vi "Alicat Simplified Driver Example.vi"() -> ()   [LabVIEW 2019]
doc: "Simplified example program for initializing the COM port, determining the data frame of an Alicat, and acquiring the data of the same Alicat.\n\nThis is intended to be a good starting point for either creating a new program or integrating Alicat devices with an existing program."
uses:
  Sub-VIs/Data Cluster.ctl
panel:
  out "Measurement Data":T1
  in  "Minimum time \nbetween readings [ms]":u32
  out "Measurements\nper second":dbl
  in  "End Program":bool
  out "Error Text":string
  out "Error Present":bool
  out "Range Exceeded":bool
  in  "COM Port Settings":T2={"Unit ID"="A", "Baud Rate"=enum."19200", "VISA Sesssion In"="COM1"}
  # "Totalizer Timer"
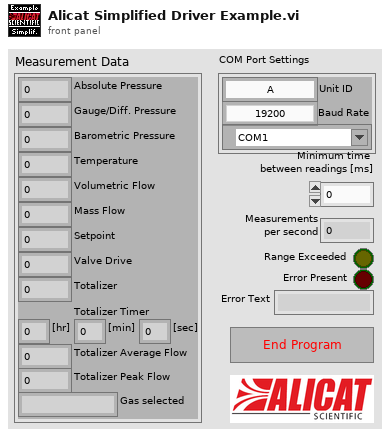
[diagram p1: front panel]
types:
  T1 = typedef "Data Cluster.ctl" = cluster{"Absolute Pressure":dbl, "Gauge/Diff. Pressure":dbl, "Barometric Pressure":dbl, "Temperature":dbl, "Volumetric Flow":dbl, "Mass Flow":dbl, "Setpoint":dbl, "Valve Drive":dbl, "Totalizer":dbl, "[hr]":dbl, "[min]":dbl, "[sec]":dbl, "Totalizer Average Flow":dbl, "Totalizer Peak Flow":dbl, "Gas selected":string}
  T2 = cluster{"Unit ID":string, "Baud Rate":enum8{"2400", "9600", "19200", "38400", "57600", "115200", "Unknown"}, "VISA Sesssion In":refnum<visa-resource-name>}
  T3 = typedef "Data Frame.ctl" = cluster{"Absolute Pressure":bool, "Gauge/Diff. Pressure":bool, "Barometric Pressure":bool, "Temperature":bool, "Volumetric":bool, "Mass":bool, "Setpoint":bool, "Valve Drive":bool, "Totalizer":bool, "Totalizer Timer":bool, "Totalizer Average Flow":bool, "Totalizer Peak Flow":bool, "Gas Selected":bool, "Tot. Timer Format":u16}
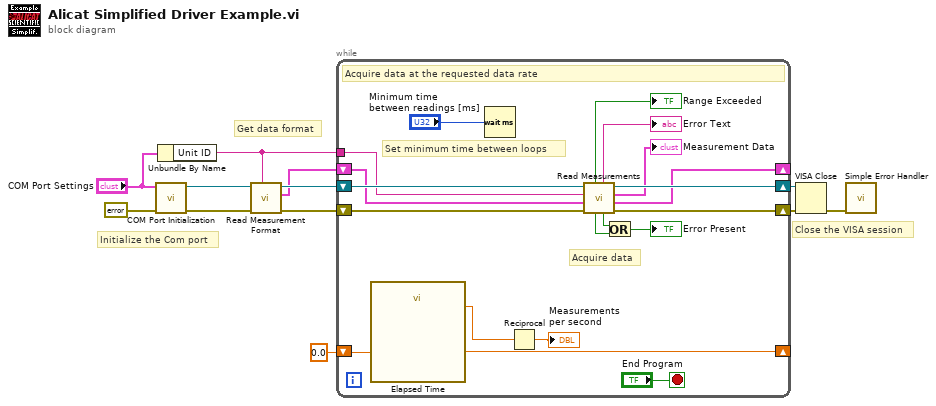
[diagram p0: block diagram]
diagram:
  # "Get data format"
  # "Close the VISA session"
  # "Initialize the Com port"
  n1 = call "COM Port Initialization.vi"("error in (no error)"=errorcluster {"status"=FALSE, "code"=0, "source"=""}, "Communication Settings"="COM Port Settings") -> ("error out"=w6:errorcluster, "VISA Session Out"=w5:refnum<visa-resource-name>)  [unwired: 8 in]
  n2 = Unbundle By Name("COM Port Settings") -> ("Unit ID"=w1:string)
  n3 = call "Read Measurement Format.vi"("Unit ID (A)"=w1, "error in"=w6, "VISA Session In"=w5) -> ("error out"=w4:errorcluster, "Data Frame Format"=w2:T3, "VISA Session Out"=w3:refnum<visa-resource-name>)  [unwired: 6 in]
  n4 = while {
    shift-right: [w28] -> _
    shift-left: 0.0 ("Set Start Time (s)") -> [w31]
    shift-right: [w26] -> w7
    shift-left: w4 -> [w30]
    shift-right: [w27] -> w8
    shift-left: w3 -> [w29]
    tunnel: w1 -> [w25]
    shift-right: [w19] -> _
    shift-left: w2 -> [w24]
    stop <- "End Program" stop-if-true
    # "Set minimum time between loops"
    # "Acquire data"
    # "Acquire data at the requested data rate"
    n5 = call "Elapsed Time"("Set Start Time (s)"=w31) -> ("Get Start Time (s)"=w28:dbl, "Elapsed Time (s)"=w15:dbl)  [unwired: 11 in, 6 out]
    n6 = Wait (ms)(milliseconds to wait="Minimum time \nbetween readings [ms]") -> ()  [unwired: 1 out]
    n7 = Reciprocal(x=w15) -> (1/x=→"Measurements\nper second":dbl)
    n8 = call "Read Measurements.vi"("error in"=w30, "Data Frame Format In"=w24, "Unit ID (A)"=w25, "VISA Session In"=w29) -> ("error out"=w26:errorcluster, "Data Frame Format Out"=w19:T3, "Data Cluster"=→"Measurement Data":T1, "VISA Session Out"=w27:refnum<visa-resource-name>, "Unknown Dataframe Info"=w23:bool, "Error/Overrange/Unknown String"=→"Error Text":string, "Error Present"=w22:bool, "Range Exceeded"=→"Range Exceeded":bool)
    n9 = Or(x=w23, y=w22) -> (x .or. y?=→"Error Present":bool)
  }
  n10 = VISA Close(VISA resource name=w8, error in (no error)=w7) -> (error out=w9:errorcluster)
  n11 = call <vilib>:"Simple Error Handler.vi"("error in (no error)"=w9) -> ()  [unwired: 4 in, 5 out]
